vi "Find Item.vi"(7 "$Path or Item Name":string, 8 "error in (no error)":errorcluster, 10 "Offset":i32, 11 "JSON":string) -> (0 "error out":errorcluster, 1 "<JSON>":string caption="<JSON>Item", 2 "Item offset":i32, 3 "Found":bool)   [LabVIEW 2017, in "JSONtext.lvlib"]
doc: "Find the JSON item at the JSON Path specified.\n\nPaths specify an item in a tree of nested Objects, and start with $.\nExample JSON:\n{\"A\":{\"A1\":123,\"A2\":4},\"B\":\"Hi\"}\nAt path $.A.A1 is 123\nAt path $.B (or just B) is \"Hi\"\nAt path $.A (or just A) is {\"A1\":123,\"A2\":4}"
uses:
  JSONtext.lvlib
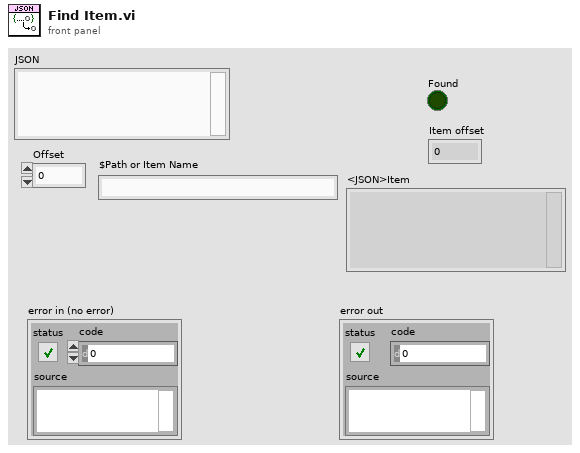
[diagram p1: front panel]
types:
  T1 = typedef "JSONtext.lvlib/Found Items.ctl" = cluster{"Item offset":i32, "Offset past Item":i32, "Name offset":i32, "Offset past Name":i32, "Found":bool, "Item Type":T2, "Item Index":i32}
  T2 = typedef "JSONtext.lvlib/Parsing State.ctl" = enum16{"Parser Error", "Object", "Array", "String", "Number/Other", "Leading Whitespace", "Object end", "Array end", "Value end"}
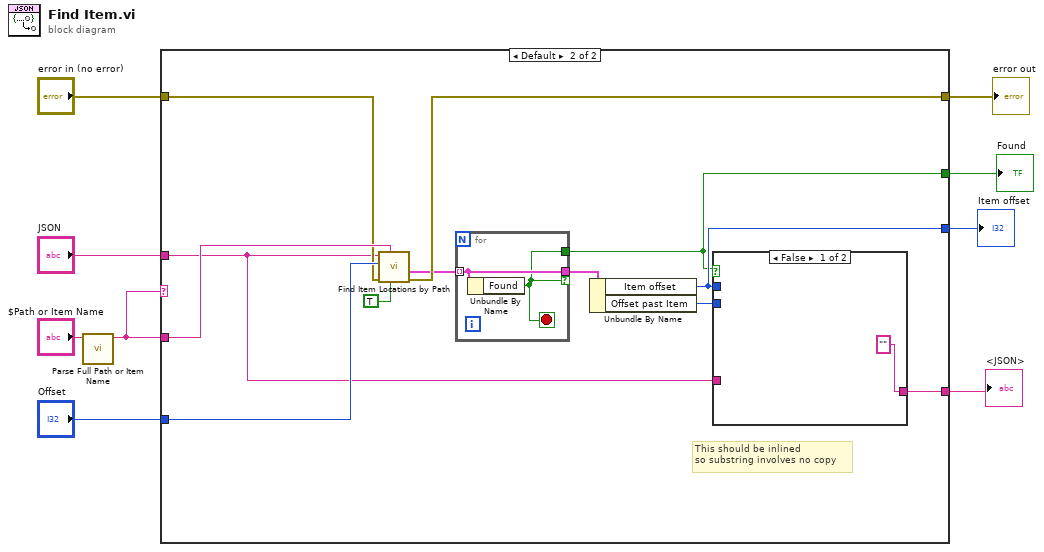
[diagram p0: block diagram]
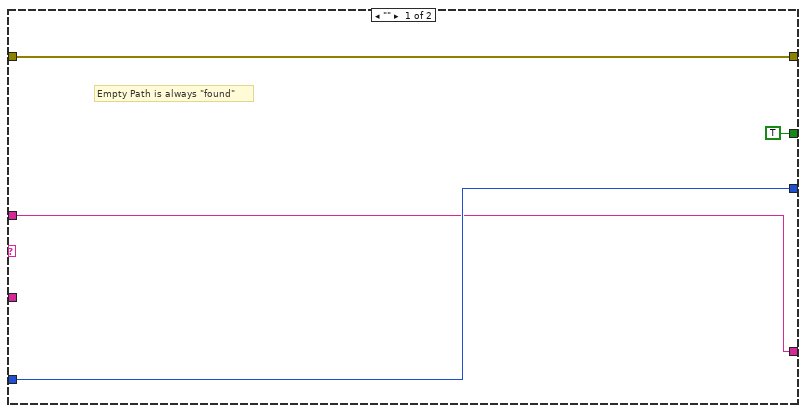
[diagram p2: hidden frame]
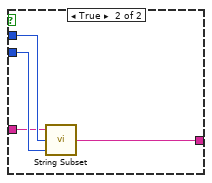
[diagram p3: hidden frame]
diagram:
  n1 = call "Parse Full Path or Item Name.vi"("Full Path (with $) or Name"="$Path or Item Name") -> ("Relative Path or JSON-format name"=w2:string)  [unwired: 10 in]
  n2 = case shown="Default" w2 {
    tunnel: w2 -> [_ w25]
    tunnel: "Offset" -> [w12 w24]
    tunnel: "error in (no error)" -> [w13 w23]
    tunnel: [w13 w22] -> w7
    tunnel: "JSON" -> [w10 w21]
    tunnel: [w12 w17] -> w5
    tunnel: [TRUE ("Found") w14] -> w4
    tunnel: [w10 w15] -> w3
    frame "" {
      # "Empty Path is always \"found\""
    }
    frame Default {
      # "This should be inlined\nso substring involves no copy"
      n3 = call "Find Item Locations by Path.vi"("Only return first found"=TRUE, "Path"=w25, "error in (no error)"=w23, "Offset"=w24, "JSON"=w21) -> ("error out"=w22:errorcluster, "Items"=w19:T1[])  [unwired: 5 in]
      n4 = for {
        tunnel: w19 -> [w27] mode=indexing
        tunnel: [w27] -> w18 if=w26
        tunnel: [w26] -> w14
        stop <- w26 stop-if-true
        n5 = Unbundle By Name(w27) -> ("Found"=w26:bool)
      }
      n6 = Unbundle By Name(w18) -> ("Item offset"=w17:i32, "Offset past Item"=w16:i32)
      n7 = case shown="False" w14 {
        tunnel: w21 -> [_ w29]
        tunnel: ["" ("substring") w32] -> w15
        tunnel: w17 -> [_ w31]
        tunnel: w16 -> [_ w30]
        frame False {
        }
        frame True {
          n8 = call "String Subset.vi"("Offset past End"=w30, "Start offset"=w31, "JSON"=w29) -> ("substring"=w32:string)  [unwired: 2 in]
        }
      }
    }
  }
  "error out" <- w7
  "<JSON>" <- w3
  "Found" <- w4
  "Item offset" <- w5
